vi "SPI Write Bits.vi"(9 "pWriteBitStr":string, 10 "SPIIndex":i32, 11 "DevHandle":i32) -> (1 "pWriteBitStr out":string, 3 "function return":i32)   [LabVIEW 2010, in "usb2spi.lvlib"]
doc: "int WINAPI SPI_WriteBits(int DevHandle,int SPIIndex,char *pWriteBitStr);"
uses:
  usb2spi.lvlib
  USB2XXX/trunk/USB2XXX/USB2XXX/vs2010/Release/USB2XXX.dll
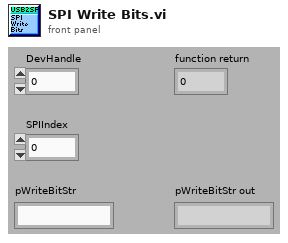
[diagram p1: front panel]
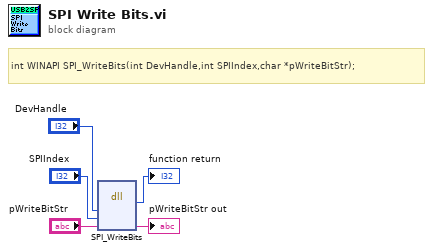
[diagram p0: block diagram]
diagram:
  # "int WINAPI SPI_WriteBits(int DevHandle,int SPIIndex,char *pWriteBitStr);"
  n1 = dll-call lib="E:/OtherWork/STM32/USB2XXX/trunk/USB2XXX/USB2XXX/vs2010/Release/USB2XXX.*" fn="SPI_WriteBits"("DevHandle"="DevHandle", "SPIIndex"="SPIIndex", "pWriteBitStr"="pWriteBitStr") -> (→"function return":i32, "pWriteBitStr"=→"pWriteBitStr out":string)  [unwired: 5 in, 2 out]
